vi "09 - viewport.vi"() -> ()   [LabVIEW 2015]
uses:
  Libraries/LibSDL2 Wrapper/Controls/Init Flags.ctl
  Libraries/LibSDL2 Wrapper/Controls/Rectangle.ctl
  Libraries/LibSDL2 Wrapper/Controls/NULL.ctl
  Libraries/LibSDL2 Wrapper/LibSDL2.lvlib
  Libraries/SDL2 Utility/SDL2 Utility.lvlib
  Libraries/LibSDL2_Image Wrapper/LibSDL2_Image.lvlib
panel:
  out "Error":string
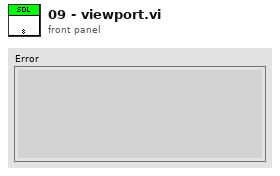
[diagram p1: front panel]
types:
  T1 = typedef "LibSDL2.lvlib/NULL.ctl" = enum32{"NULL"}
  T2 = typedef "LibSDL2.lvlib/Rectangle.ctl" = cluster{"x":i32, "y":i32, "Width":i32, "Height":i32}
  T3 = typedef "LibSDL2.lvlib/Init Flags.ctl" = u32
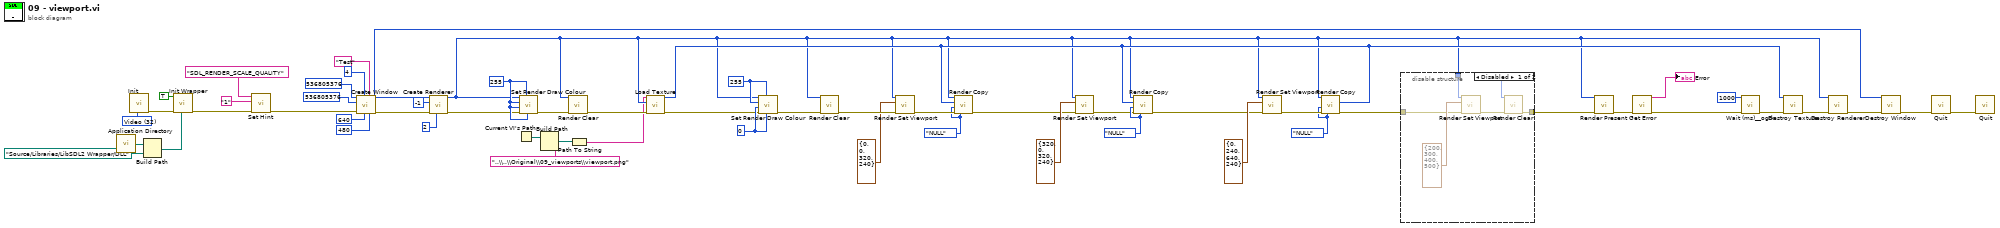
[diagram p0: block diagram]
diagram:
  w13 = NULL."NULL" ("Null")
  w19 = NULL."NULL" ("Null")
  w20 = NULL."NULL" ("Null")
  w34 = u8 0 ("B")
  w35 = u8 255 ("R")
  w41 = u8 255 ("R")
  w57 = T3 32 items=["Timer"=1, "Audio"=16, "Video"=32, "Joystick"=512, "Haptic"=4096, "Game Controller"=8192, "Events"=16384, "No Parachute"=1048576, "Everything"=17244689] ("Init Flags")
  n1 = call <vilib>:"Application Directory.vi"() -> ("Application Directory"=w6:path)
  n2 = call "Init.vi"("Flags"=w57) -> ("error out"=w31:errorcluster)  [unwired: 9 in, 1 out]
  n3 = Build Path(base path=w6, name or relative path=path "Source/Libraries/LibSDL2 Wrapper/DLL" ("DLL Directory")) -> (appended path=w5:path)
  n4 = call "Init Wrapper.vi"("DLL Directory"=w5, "error in"=w31, "PNG (F)"=TRUE) -> ("error out"=w30:errorcluster)  [unwired: 7 in, 1 out]
  n5 = call "Set Hint.vi"("error in"=w30, "Value"="1", "Name"="SDL_RENDER_SCALE_QUALITY") -> ("error out"=w48:errorcluster)  [unwired: 7 in, 1 out]
  n6 = call "Create Window.vi"("Height"=480, "Title"="Test", "Width"=640, "Flags"=u32 4, "error in"=w48, "Position y"=u32 536805376 ("Flags"), "Position x"=u32 536805376 ("Flags")) -> ("error out"=w45:errorcluster, "Window Pointer"=w44:u32)  [unwired: 3 in]
  n7 = call "Create Renderer.vi"("Flags"=u32 2, "error in"=w45, "Index"=-1, "Window Pointer"=w44) -> ("error out"=w39:errorcluster, "Renderer Pointer"=w9:u32)  [unwired: 6 in]
  n8 = Current VI's Path() -> (path=w2:path)
  n9 = call "Set Render Draw Colour.vi"("B"=w41, "A"=w41, "error in (no error)"=w39, "G"=w41, "R"=w41, "Renderer Pointer"=w9) -> ("error out"=w36:errorcluster)  [unwired: 4 in, 1 out]
  n10 = Build Path(base path=w2, name or relative path="..\\..\\Original\\09_viewports\\viewport.png" ("File")) -> (appended path=w3:path)
  n11 = call "Render Clear.vi"("error in"=w36, "Renderer Pointer"=w9) -> ("error out"=w33:errorcluster)  [unwired: 8 in, 1 out]
  n12 = Path To String(path=w3) -> (string=w1:string)
  n13 = call "Load Texture.vi"("error in"=w33, "Renderer Pointer"=w9, "File"=w1) -> ("error out"=w32:errorcluster, "Optimised Texture Pointer"=w11:u32)  [unwired: 5 in, 2 out]
  n14 = call "Set Render Draw Colour.vi"("B"=w34, "A"=w35, "error in (no error)"=w32, "G"=w34, "R"=w35, "Renderer Pointer"=w9) -> ("error out"=w24:errorcluster)  [unwired: 4 in, 1 out]
  n15 = call "Render Clear.vi"("error in"=w24, "Renderer Pointer"=w9) -> ("error out"=w23:errorcluster)  [unwired: 8 in, 1 out]
  n16 = call "Render Set Viewport.vi"("error in"=w23, "Rectangle"=T2 {"x"=0, "y"=0, "Width"=320, "Height"=240}, "Renderer Pointer"=w9) -> ("error out"=w21:errorcluster)  [unwired: 7 in, 1 out]
  n17 = call "Render Copy.vi"("Destination Rectangle Pointer"=w20, "error in"=w21, "Source Rectangle Pointer"=w20, "Texture Pointer"=w11, "Renderer Pointer"=w9) -> ("error out"=w16:errorcluster)  [unwired: 5 in, 1 out]
  n18 = call "Render Set Viewport.vi"("error in"=w16, "Rectangle"=T2 {"x"=320, "y"=0, "Width"=320, "Height"=240}, "Renderer Pointer"=w9) -> ("error out"=w18:errorcluster)  [unwired: 7 in, 1 out]
  n19 = call "Render Copy.vi"("Destination Rectangle Pointer"=w19, "error in"=w18, "Source Rectangle Pointer"=w19, "Texture Pointer"=w11, "Renderer Pointer"=w9) -> ("error out"=w12:errorcluster)  [unwired: 5 in, 1 out]
  n20 = call "Render Set Viewport.vi"("error in"=w12, "Rectangle"=T2 {"x"=0, "y"=240, "Width"=640, "Height"=240}, "Renderer Pointer"=w9) -> ("error out"=w14:errorcluster)  [unwired: 7 in, 1 out]
  n21 = call "Render Copy.vi"("Destination Rectangle Pointer"=w13, "error in"=w14, "Source Rectangle Pointer"=w13, "Texture Pointer"=w11, "Renderer Pointer"=w9) -> ("error out"=w10:errorcluster)  [unwired: 5 in, 1 out]
  n22 = disable-structure shown="Disabled" {
    disable-tunnel: w10 -> [w61 w63]
    disable-tunnel: w9 -> [w59 _]
    disable-tunnel: [w58 w63] -> w8
    frame Disabled {
      n23 = call "Render Set Viewport.vi"("error in"=w61, "Rectangle"=T2 {"x"=200, "y"=300, "Width"=400, "Height"=500}, "Renderer Pointer"=w59) -> ("error out"=w60:errorcluster)  [unwired: 7 in, 1 out]
      n24 = call "Render Clear.vi"("error in"=w60, "Renderer Pointer"=w59) -> ("error out"=w58:errorcluster)  [unwired: 8 in, 1 out]
    }
    frame Enabled {
    }
  }
  n25 = call "Render Present.vi"("error in"=w8, "Renderer Pointer"=w9) -> ("error out"=w38:errorcluster)  [unwired: 9 in]
  n26 = call "Get Error.vi"("error in"=w38) -> ("error out"=w37:errorcluster, "Error"=→"Error":string)  [unwired: 9 in]
  n27 = call <userlib>:"Wait (ms)__ogtk.vi"("error in (no error)"=w37, "milliseconds to wait"=u32 1000) -> ("error out"=w26:errorcluster)  [unwired: 8 in, 1 out]
  n28 = call "Destroy Texture.vi"("error in"=w26, "Texture Pointer"=w11) -> ("error out"=w25:errorcluster)  [unwired: 9 in]
  n29 = call "Destroy Renderer.vi"("error in"=w25, "Renderer Pointer"=w9) -> ("error out"=w40:errorcluster)  [unwired: 9 in]
  n30 = call "Destroy Window.vi"("error in"=w40, "Window Pointer"=w44) -> ("error out"=w28:errorcluster)  [unwired: 9 in]
  n31 = call "Quit.vi"("error in"=w28) -> ("error out"=w27:errorcluster)  [unwired: 10 in]
  n32 = call "Quit.vi"("error in"=w27) -> ()  [unwired: 10 in, 1 out]
